vi "Overlay Image.vi"(8 "error in":errorcluster, 9 "String in":string, 10 "Enum":T2, 11 "path in":path) -> (0 "error out":errorcluster, 2 "String out":string, 3 "image data":T1)   [LabVIEW 2013, in "configuration library.lvlib"]
uses:
  configuration library.lvlib
  Configuration Editor/subVIs/Glyphs Status.ctl
  <vilib>/picture/picture.llb/imagedata.ctl
  Configuration Editor/PL Framework Configuration Tool.lvlib
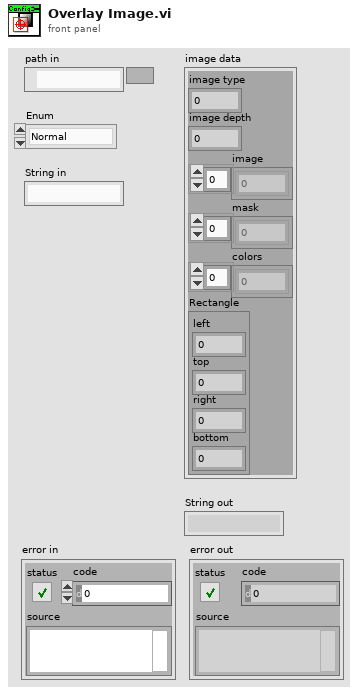
[diagram p1: front panel]
types:
  T1 = typedef "imagedata.ctl" = cluster{"image type":i32, "image depth":i32, "image":u8[], "mask":u8[], "colors":u32[], "Rectangle":cluster{"left":i16, "top":i16, "right":i16, "bottom":i16}}
  T2 = typedef "PL Framework Configuration Tool.lvlib/Glyphs Status.ctl" = enum16{"Normal", "Error", "Async"}
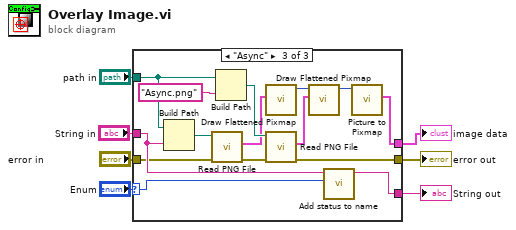
[diagram p0: block diagram]
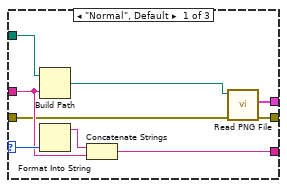
[diagram p2: hidden frame]
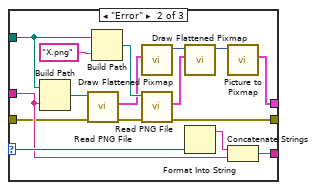
[diagram p3: hidden frame]
diagram:
  n1 = case shown="\"Async\"" "Enum" {
    selector: "Enum" -> [w13 w23 w38]
    tunnel: "path in" -> [w16 w24 w39]
    tunnel: [w14 w27 w42] -> w4
    tunnel: "String in" -> [w11 w22 w37]
    tunnel: [w10 w20 w36] -> w6
    tunnel: "error in" -> [w9 w19 w35]
    tunnel: [w8 w17 w33] -> w1
    frame "Normal", Default {
      n2 = Build Path(base path=w16, name or relative path=w11) -> (appended path=w15:path)
      n3 = Format Into String(w13) -> (resulting string=w12:string)  [unwired: 3 in, 1 out]
      n4 = Concatenate Strings(w12, w11) -> (w10:string)
      n5 = call <vilib>:"Read PNG File.vi"("error in (no error)"=w9, "path to PNG file"=w15) -> ("error out"=w8:errorcluster, "image data"=w14:T1)  [unwired: 7 in, 1 out]
    }
    frame "Error" {
      n6 = Build Path(base path=w24, name or relative path=w22) -> (appended path=w32:path)
      n7 = call <vilib>:"Read PNG File.vi"("error in (no error)"=w19, "path to PNG file"=w32) -> ("error out"=w18:errorcluster, "image data"=w28:T1)  [unwired: 7 in, 1 out]
      n8 = Build Path(base path=w24, name or relative path="X.png") -> (appended path=w30:path)
      n9 = call <vilib>:"Draw Flattened Pixmap.vi"("image data"=w28) -> ("new picture"=w26:picture)  [unwired: 8 in]
      n10 = call <vilib>:"Read PNG File.vi"("error in (no error)"=w18, "path to PNG file"=w30) -> ("error out"=w17:errorcluster, "image data"=w25:T1)  [unwired: 7 in, 1 out]
      n11 = call <vilib>:"Draw Flattened Pixmap.vi"("image data"=w25, "picture"=w26) -> ("new picture"=w29:picture)  [unwired: 7 in]
      n12 = Format Into String(w23) -> (resulting string=w21:string)  [unwired: 3 in, 1 out]
      n13 = call <vilib>:"Picture to Pixmap.vi"("picture"=w29) -> ("image data"=w27:T1)  [unwired: 9 in, 1 out]
      n14 = Concatenate Strings(w21, w22) -> (w20:string)
    }
    frame "Async" {
      n15 = Build Path(base path=w39, name or relative path=w37) -> (appended path=w47:path)
      n16 = call <vilib>:"Read PNG File.vi"("error in (no error)"=w35, "path to PNG file"=w47) -> ("error out"=w34:errorcluster, "image data"=w43:T1)  [unwired: 7 in, 1 out]
      n17 = Build Path(base path=w39, name or relative path="Async.png") -> (appended path=w45:path)
      n18 = call <vilib>:"Draw Flattened Pixmap.vi"("image data"=w43) -> ("new picture"=w41:picture)  [unwired: 8 in]
      n19 = call <vilib>:"Read PNG File.vi"("error in (no error)"=w34, "path to PNG file"=w45) -> ("error out"=w33:errorcluster, "image data"=w40:T1)  [unwired: 7 in, 1 out]
      n20 = call <vilib>:"Draw Flattened Pixmap.vi"("image data"=w40, "picture"=w41) -> ("new picture"=w44:picture)  [unwired: 7 in]
      n21 = call "Add status to name.vi"("Status"=w38, "Name"=w37) -> ("Name with status"=w36:string)  [unwired: 9 in]
      n22 = call <vilib>:"Picture to Pixmap.vi"("picture"=w44) -> ("image data"=w42:T1)  [unwired: 9 in, 1 out]
    }
  }
  "String out" <- w6
  "image data" <- w4
  "error out" <- w1
